vi "Setup Facade Controls.vi"(8 "Progress Bar Refnum":refnum<vi>, 9 "Glyph Refnum":refnum<vi>, 10 "State":T1={"Window Handle"=refnum, "Maximum"=100, "State Change Action"=enum."No Action", "Running"=FALSE, "Visable Items"={"Label"=TRUE, "Caption"=FALSE}, "Value"=0, "Show Progress Bar"=FALSE}, 11 "Container State":T3) -> ()   [LabVIEW 2011, in "Taskbar Progress Bar.xctl"]
uses:
  Taskbar Progress Bar.xctl
  <vilib>/_xctls/Container State.ctl
  Abilities/PB State.ctl
  TypeDefs/Dispaly State Change Methods.ctl
  <vilib>/Utility/miscctls.llb/LVPositionTypeDef.ctl
  <vilib>/Utility/miscctls.llb/LVBoundsTypeDef.ctl
  <vilib>/_xctls/XControlSupport.lvlib
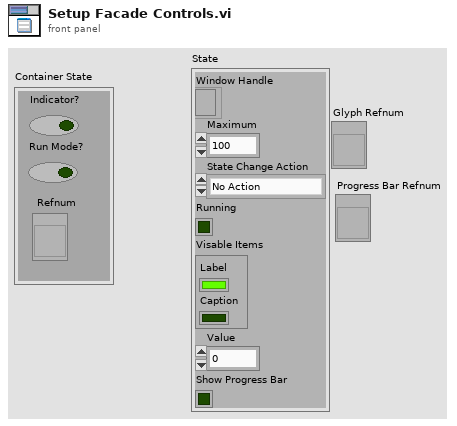
[diagram p1: front panel]
types:
  T1 = typedef "Taskbar Progress Bar.xctl/PB State.ctl" = cluster{"Window Handle":refnum<k24>, "Maximum":u64, "State Change Action":T2, "Running":bool, "Visable Items":cluster{"Label":bool, "Caption":bool}, "Value":u64, "Show Progress Bar":bool}
  T2 = typedef "Taskbar Progress Bar.xctl/Dispaly State Change Methods.ctl" = enum16{"No Action", "Created", "Method - Initialize", "Method - Increment", "Method - Pause", "Method - Error", "Method - Finish", "Property - Show Progress Bar"}
  T3 = typedef "XControlSupport.lvlib/Container State.ctl" = cluster{"Indicator?":bool, "Run Mode?":bool, " Refnum":refnum<vi>}
  T4 = typedef "LVBoundsTypeDef.ctl" = cluster{"Width":u32, "Height":u32}
  T5 = typedef "LVPositionTypeDef.ctl" = cluster{"Left":i32, "Top":i32}
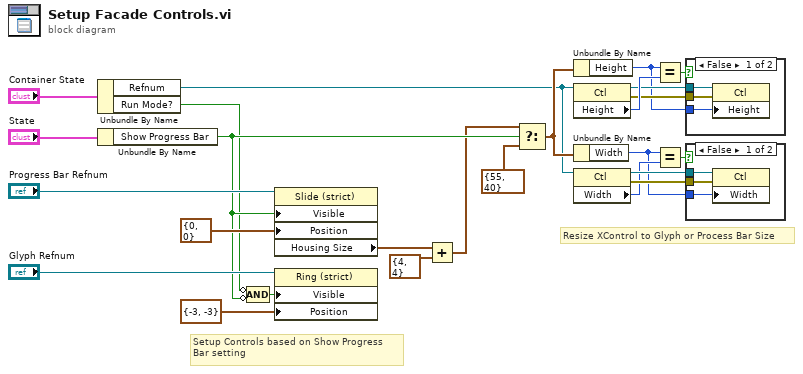
[diagram p0: block diagram]
diagram:
  # "Resize XControl to Glyph or Process Bar Size"
  # "Setup Controls based on Show Progress\nBar setting"
  n1 = Unbundle By Name("Container State") -> ("Refnum"=w5:refnum<vi>, "Run Mode?"=w6:bool)
  n2 = Unbundle By Name("State") -> ("Show Progress Bar"=w7:bool)
  n3 = Compound Arithmetic op=AND(invert w6, invert w7) -> (w4:bool)
  n4 = property class="Slide (strict)"(reference="Progress Bar Refnum", "Visible"=w7, "Position"=T5 {"Left"=0, "Top"=0}) -> ("Housing Size"=w10:T4)  [unwired: 1 in, 2 out]
  n5 = property class="Ring (strict)"(reference="Glyph Refnum", "Visible"=w4, "Position"=T5 {"Left"=-3, "Top"=-3}) -> ()  [unwired: 1 in, 2 out]
  n6 = Add(x=w10, y=T4 {"Width"=4, "Height"=4}) -> (x+y=w2:T4)
  n7 = Select(t=w2, s=w7, f=T4 {"Width"=55, "Height"=40} ("input cluster")) -> (s? t:f=w8:T4)
  n8 = Unbundle By Name(w8) -> ("Height"=w11:u32)
  n9 = property class="Ctl"(reference=w5) -> (reference out=w12:refnum<vi>, error out=w13:errorcluster, "Height"=w14:u32)  [unwired: 1 in]
  n10 = Unbundle By Name(w8) -> ("Width"=w9:u32)
  n11 = property class="Ctl"(reference=w5) -> (reference out=w19:refnum<vi>, error out=w18:errorcluster, "Width"=w17:u32)  [unwired: 1 in]
  n12 = Equal?(x=w11, y=w14) -> (x = y?=w15:bool)
  n13 = Equal?(x=w9, y=w17) -> (x = y?=w16:bool)
  n14 = case shown="False" w15 {
    tunnel: w12 -> [w28 _]
    tunnel: w13 -> [w27 _]
    tunnel: w11 -> [w26 _]
    frame False {
      n15 = property class="Ctl"(reference=w28, error in=w27, "Height"=w26) -> ()  [unwired: 2 out]
    }
    frame True {
    }
  }
  n16 = case shown="False" w16 {
    tunnel: w19 -> [w31 _]
    tunnel: w18 -> [w30 _]
    tunnel: w9 -> [w29 _]
    frame False {
      n17 = property class="Ctl"(reference=w31, error in=w30, "Width"=w29) -> ()  [unwired: 2 out]
    }
    frame True {
    }
  }
